vi "BLE_Sample - Test.vi"() -> (2 "Table Control":string[][](table))   [LabVIEW 2020]
uses:
  C:/Users/Kevin/Desktop/BLE/BLELib.dll
  BLELib.dll
panel:
  out "DisConnect_BLE_ByAddress":bool
  out "Numeric 2":i32
  out "Manf_ID":string[](array[string])
  out "Numeric":i32
  out "BluetoothAddress":string[][](array[string])
  out "Scanning":string
  out "error out":errorcluster
  out "Pair Result":string
  in  "stop scan":bool
  out "StoptDeviceWatcher":string
  out "StartDeviceWatcher":string
  # "A4:DA:32:0D:F5:E2"
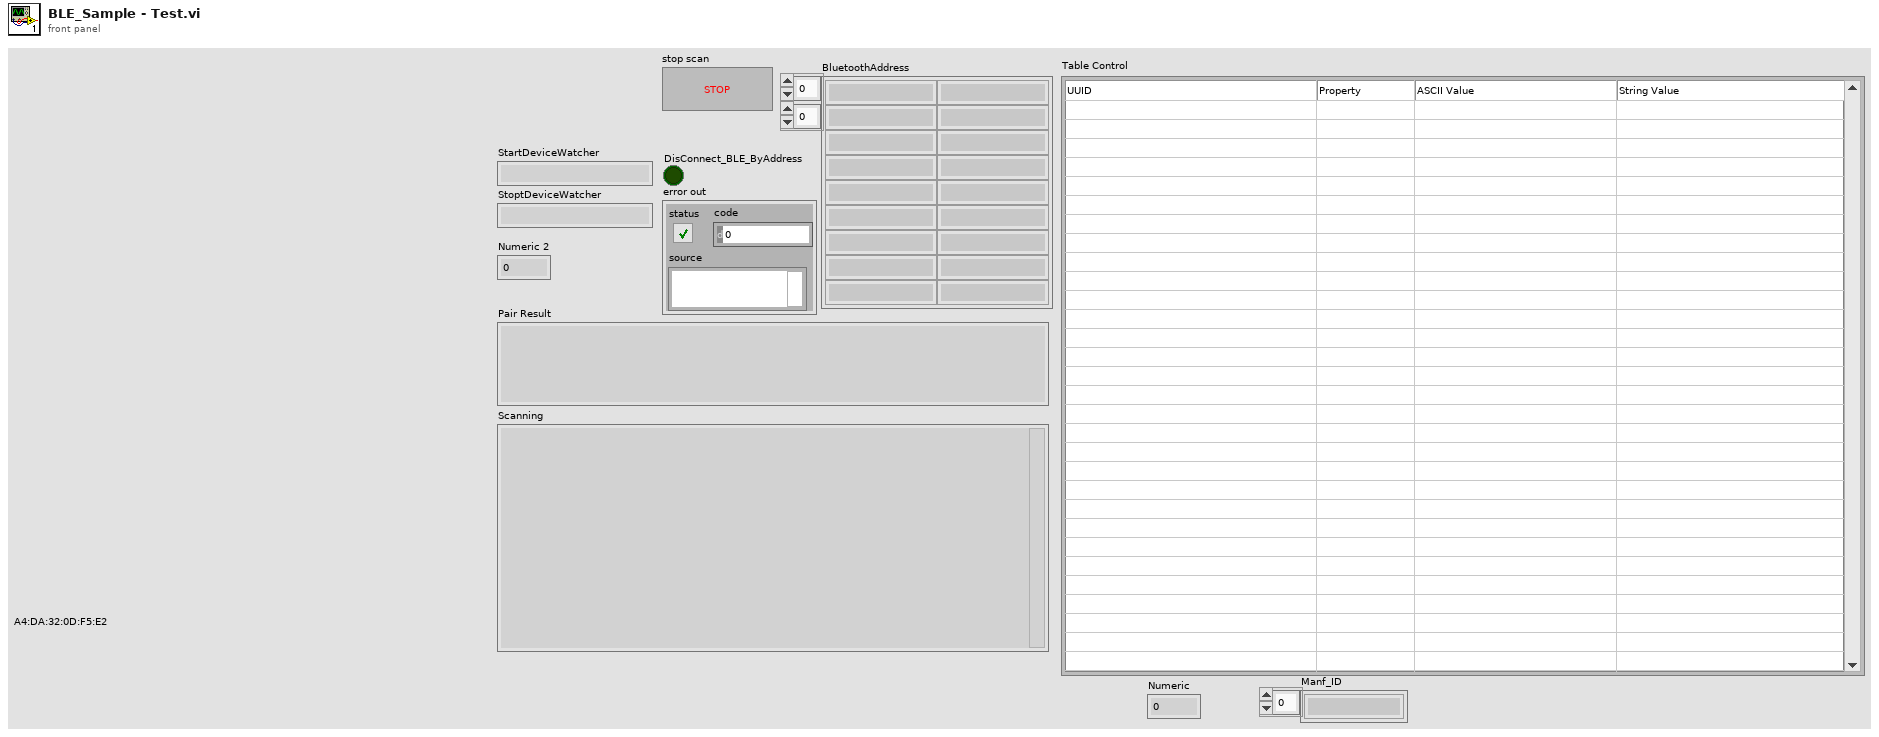
[diagram p1: front panel]
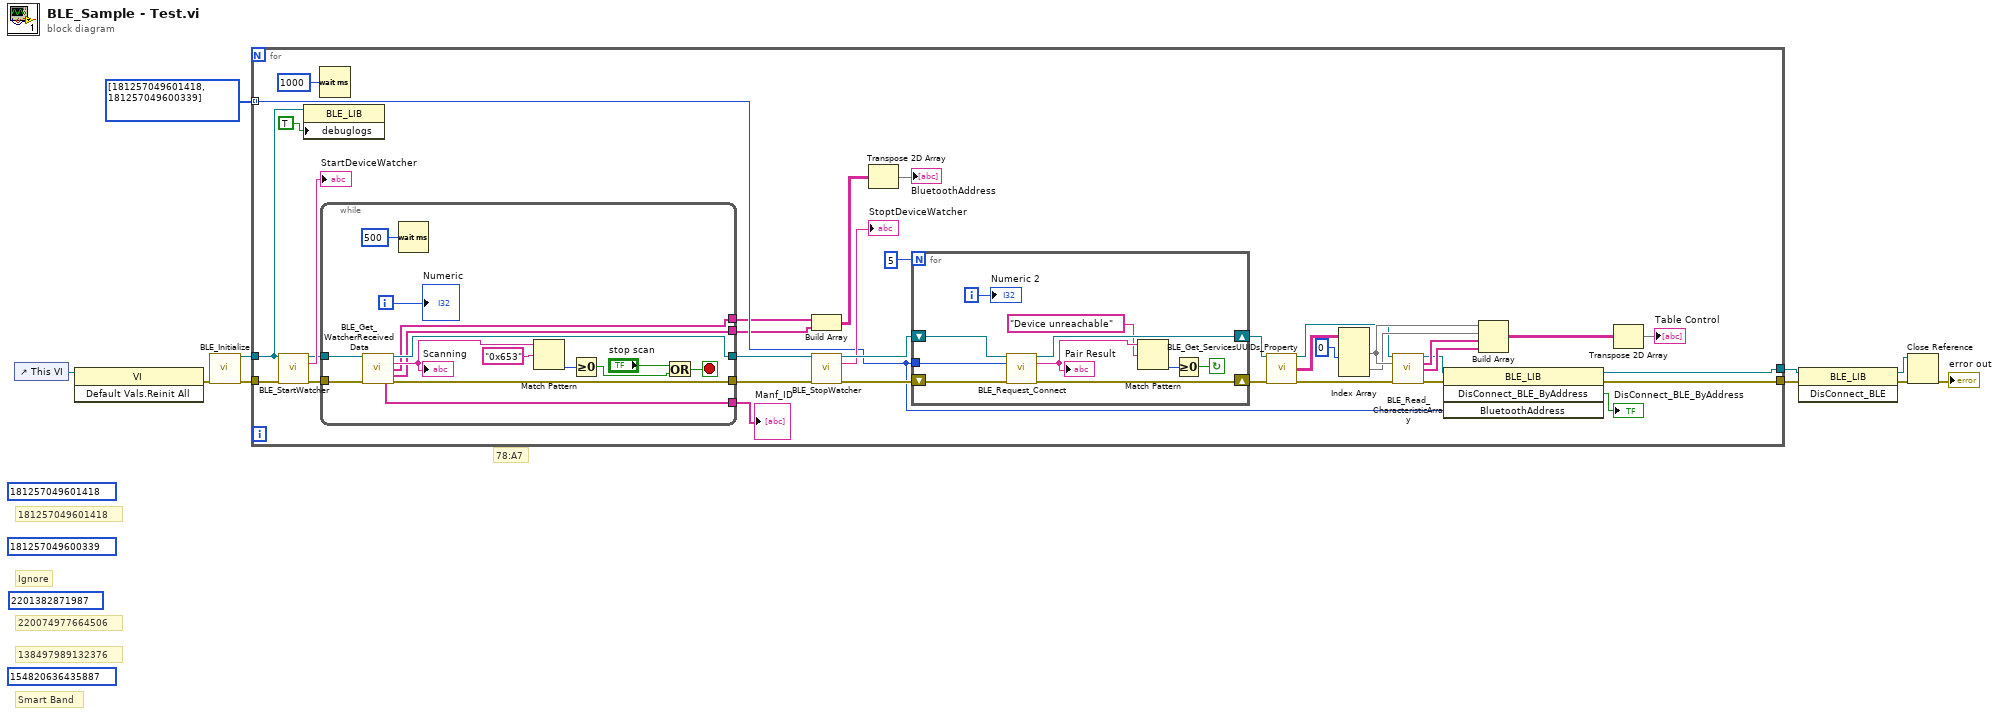
[diagram p0: block diagram]
diagram:
  (unwired) u64 181257049600339 ("BluetoothAddress")
  (unwired) u64 2201382871987 ("BluetoothAddress")
  (unwired) u64 154820636435887 ("BluetoothAddress")
  (unwired) u64 181257049601418 ("BluetoothAddress")
  # "138497989132376"
  # "220074977664506"
  # "Ignore"
  # "78:A7"
  # "181257049601418"
  # "Smart Band"
  n1 = control-ref of="This VI"() -> (w10:refnum<vi>)
  n2 = invoke class="VI" method="Default Vals.Reinit All"(reference=w10) -> (error out=w8:errorcluster)  [unwired: 2 in, 2 out]
  n3 = call "BLE_Initialize.vi"("error in (no error)"=w8) -> (".NET Refnum out"=w6:refnum<k24>, "error out"=w7:errorcluster)  [unwired: 13 in]
  n4 = for {
    tunnel: [w22] -> w4
    tunnel: w6 -> [w41]
    tunnel: w7 -> [w40]
    tunnel: u64[] [181257049601418, 181257049600339] -> [w24] mode=indexing
    tunnel: [w21] -> w2
    n5 = call "BLE_StartWatcher.vi"(".NET Refnum in"=w41, "error in (no error)"=w40) -> (".NET Refnum out"=w16:refnum<k24>, "StartDeviceWatcher"=→"StartDeviceWatcher":string, "error out"=w18:errorcluster)  [unwired: 11 in]
    n6 = property class="BLE_LIB"(reference=w41, "debuglogs"=TRUE) -> ()  [unwired: 1 in, 2 out]
    n7 = Wait (ms)(milliseconds to wait=u32 1000) -> ()  [unwired: 1 out]
    n8 = while {
      tunnel: [w51] -> w15
      tunnel: w16 -> [w55]
      tunnel: [w52] -> w14
      tunnel: w18 -> [w53]
      tunnel: [w50] -> w13
      tunnel: [w49] -> w12
      tunnel: [w47] -> w11
      i -> [w48]
      stop <- w56 stop-if-true
      n9 = call "BLE_Get_WatcherReceivedData.vi"(".NET Refnum in"=w55, "error in (no error)"=w53) -> (".NET Refnum out"=w51:refnum<k24>, "Watcher Response"=w54:string, "Bluetooth Addr"=w50:string[], "Bluetooth Raw Addr"=w49:string[], "Manf_ID"=w47:string[], "error out"=w52:errorcluster)  [unwired: 6 in, 2 out]
      "Scanning" <- w54
      n10 = Wait (ms)(milliseconds to wait=u32 500) -> ()  [unwired: 1 out]
      n11 = Match Pattern(string=w54, regular expression="0x653") -> (offset past match=w59:i32)  [unwired: 1 in, 3 out]
      n12 = Greater Or Equal To 0?(x=w59) -> (x >= 0?=w57:bool)
      n13 = Or(x="stop scan", y=w57) -> (x .or. y?=w56:bool)
      "Numeric" <- w48
    }
    "Manf_ID" <- w11
    n14 = Build Array(w13, w12) -> (w44:string[][])
    n15 = call "BLE_StopWatcher.vi"(".NET Refnum in"=w15, "error in (no error)"=w14) -> (".NET Refnum out"=w45:refnum<k24>, "StoptDeviceWatcher"=→"StoptDeviceWatcher":string, "error out"=w46:errorcluster)  [unwired: 11 in]
    n16 = Transpose 2D Array(2D array=w44) -> (transposed array=→"BluetoothAddress":string[][])
    n17 = for {
      N: 5 -> [_]
      tunnel: w24 -> [w69]
      shift-right: [w67] -> w37
      shift-left: w46 -> [w71]
      shift-right: [w68] -> w38
      shift-left: w45 -> [w70]
      i -> [w62]
      stop <- w63 continue-if-true
      n18 = call "BLE_Request_Connect.vi"(".NET Refnum in"=w70, "BluetoothAddress"=w69, "error in (no error)"=w71) -> (".NET Refnum out"=w68:refnum<k24>, "ConnectBLE"=w66:string, "error out"=w67:errorcluster)  [unwired: 10 in]
      "Pair Result" <- w66
      n19 = Match Pattern(string=w66, regular expression="Device unreachable") -> (offset past match=w64:i32)  [unwired: 1 in, 3 out]
      n20 = Greater Or Equal To 0?(x=w64) -> (x >= 0?=w63:bool)
      "Numeric 2" <- w62
    }
    n21 = call "BLE_Get_ServicesUUIDs_Property.vi"(".NET Refnum in"=w38, "error in (no error)"=w37) -> (".NET Refnum out"=w26:refnum<k24>, "Char Val-Property"=w28:string[][], "error out"=w27:errorcluster)  [unwired: 11 in]
    n22 = Index Array(array=w28, index (col) #1=0 ("disabled index (col)")) -> (element #1=w31:string[], element #2=w30:string[])  [unwired: 3 in]
    n23 = call "BLE_Read_CharacteristicArray.vi"(".NET Refnum in"=w26, "ServicesUUIDs Extract Value"=w31, "error in (no error)"=w27) -> (".NET Refnum out"=w23:refnum<k24>, "ServicesUUIDs ASCII Value"=w35:string[], "ServicesUUIDs Value"=w34:string[], "error out"=w20:errorcluster)  [unwired: 9 in]
    n24 = invoke class="BLE_LIB" method="DisConnect_BLE_ByAddress"(reference=w23, error in=w20, "BluetoothAddress"=w24) -> (reference out=w22:refnum<k24>, error out=w21:errorcluster, "DisConnect_BLE_ByAddress"=→"DisConnect_BLE_ByAddress":bool)  [unwired: 1 in, 1 out]
    n25 = Build Array(w31, w30, w35, w34) -> (w33:string[][])
    n26 = Transpose 2D Array(2D array=w33) -> (transposed array=→"Table Control":string[][])
  }
  n27 = invoke class="BLE_LIB" method="DisConnect_BLE"(reference=w4, error in=w2) -> (reference out=w3:refnum<k24>, error out=w1:errorcluster)  [unwired: 1 in, 1 out]
  n28 = Close Reference(reference=w3, error in (no error)=w1) -> (error out=→"error out":errorcluster)
